vi "Initialize.vi"(6 "iName":string, 7 "iType":string, 8 "error in (no error)":errorcluster, 11 "Application Data":path) -> (0 "error out":errorcluster, 3 "Assembler out":refnum<class "Assembler.lvclass">)   [LabVIEW 2016, in "CLD Exam - Car Wash.lvlib" / "Assembler.lvclass"]
uses:
  Assembler.lvclass
  D:/Repos/Stream/software/Actor/Actor Class/Ancestral Actor.lvclass
  Actor/Actor Class/Ancestral Actor.lvclass/Ancestral Actor.ctl
  Assembler.lvclass/Assembler.ctl
  Actor/Actor Class/Ancestral Actor.lvclass
  Mediator/Classes/Message Broker Interface Ref/Message Broker Interface Ref.lvclass
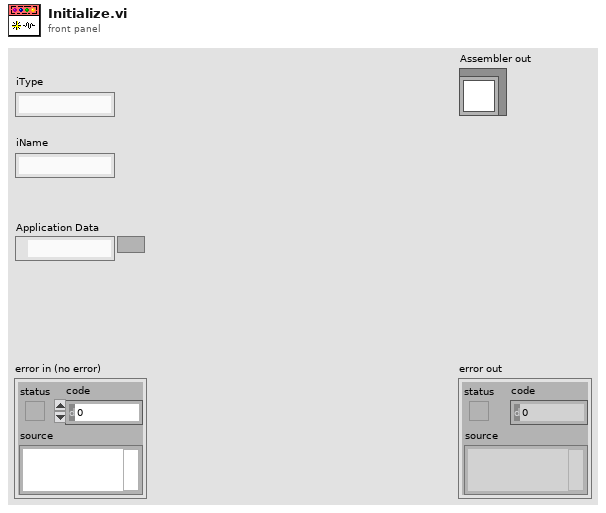
[diagram p1: front panel]
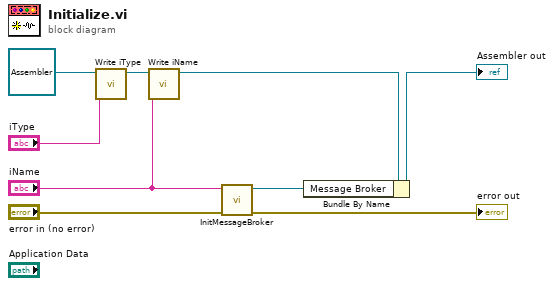
[diagram p0: block diagram]
diagram:
  n1 = call "Write iType.vi"("iType"="iType", "Ancestral Actor in"=refnum<class "Assembler.lvclass"> refnum ("Assembler in")) -> ("Ancestral Actor out"=w8:refnum<class "Assembler.lvclass">)  [unwired: 8 in, 1 out]
  n2 = call "Write iName.vi"("iName"="iName", "Ancestral Actor in"=w8) -> ("Ancestral Actor out"=w2:refnum<class "Assembler.lvclass">)  [unwired: 8 in, 1 out]
  n3 = call "InitMessageBroker.vi"("error in (no error)"="error in (no error)", "Broker Name"="iName") -> ("error out"=→"error out":errorcluster, "Message Broker Interface Ref out"=w3:refnum<class "Message Broker Interface Ref.lvclass">)  [unwired: 8 in]
  n4 = Bundle By Name(cluster=w2, "Message Broker"=w3) -> (→"Assembler out":refnum<class "Assembler.lvclass">)
